vi "Create.vi"(8 "error in (no error)":errorcluster, 9 "EventDataUserEvent":refnum<user-event>, 10 "EventData":refnum<class "EventData.lvclass">) -> (0 "error out":errorcluster, 3 "Event out":refnum<class "Event.lvclass">)   [LabVIEW 2021, in "EventManagerLibrary.lvlib" / "Event.lvclass"]
doc: "Creates an Event object with an EventToken. The user event must be valid at the time this vi executes.\n\nReturns error 510301 if the User Event reference number is zero.\nReturns error 510302 if the User Event has been previously destroyed."
uses:
  Event.lvclass
  EventDataObject/EventData.lvclass
  EventToken/EventToken.lvclass
  EventManagerErrors/EventManagerErrors.lvclass
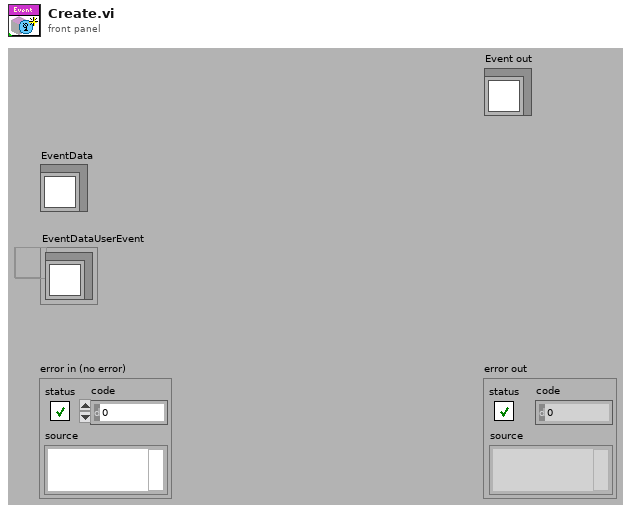
[diagram p1: front panel]
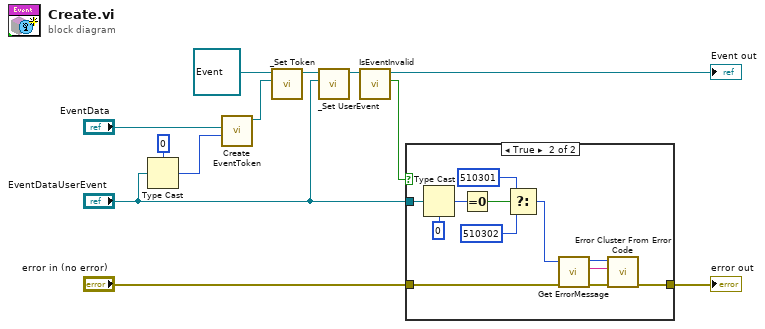
[diagram p0: block diagram]
diagram:
  n1 = Type Cast(type=0, x="EventDataUserEvent") -> (*(type *) &x=w7:i32)
  n2 = call "Create EventToken.vi"("EventRefnum"=w7, "EventData Class"="EventData") -> ("EventToken out"=w9:refnum<class "EventToken.lvclass">)  [unwired: 1 in, 8 out]
  n3 = call "_Set Token.vi"("EventToken"=w9, "Event in"=refnum<class "Event.lvclass"> refnum) -> ("Event out"=w11:refnum<class "Event.lvclass">)  [unwired: 1 in, 8 out]
  n4 = call "_Set UserEvent.vi"("UserEvent"="EventDataUserEvent", "Event in"=w11) -> ("Event out"=w6:refnum<class "Event.lvclass">)  [unwired: 9 out]
  n5 = call "IsEventInvalid.vi"("Event in"=w6) -> ("Invalid Event?"=w5:bool, "Event out"=→"Event out":refnum<class "Event.lvclass">)  [unwired: 1 in, 8 out]
  n6 = case shown="True" w5 {
    tunnel: "error in (no error)" -> [w13 w16]
    tunnel: "EventDataUserEvent" -> [_ w24]
    tunnel: [w13 w14] -> w1
    frame False {
    }
    frame True {
      n7 = Type Cast(type=0, x=w24) -> (*(type *) &x=w21:i32)
      n8 = Equal To 0?(x=w21) -> (x = 0?=w20:bool)
      n9 = Select(t=510301 ("error code (0)"), s=w20, f=510302 ("error code (0)")) -> (s? t:f=w17:i32)
      n10 = call "Get ErrorMessage.vi"("error in (no error)"=w16, "Error Code"=w17) -> ("error out"=w15:errorcluster, "Error Message"=w23:string, "Error Code"=w22:i32)  [unwired: 7 in]
      n11 = call <vilib>:"Error Cluster From Error Code.vi"("error in (no error)"=w15, "error message (\"\")"=w23, "error code (0)"=w22) -> ("error out"=w14:errorcluster)  [unwired: 1 in, 5 out]
    }
  }
  "error out" <- w1
